vi "Global 3.vi"() -> ()   [LabVIEW 2009]
panel:
  in  "Numeric":dbl
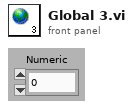
[diagram p1: front panel]
diagram:
